vi "配置初始化.vi"(8 "error in (no error)":errorcluster) -> (0 "error out":errorcluster)   [LabVIEW 2016, in "斯坦道总氮.lvlib"]
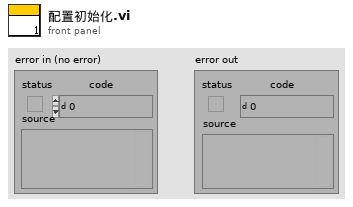
[diagram p1: front panel]
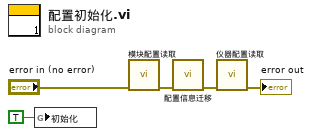
[diagram p0: block diagram]
diagram:
  n1 = global write "VAR总磷总氮全局变量.vi" "初始化"(TRUE ("内部初始化")) -> ()
  n2 = call "模块配置读取.vi"("error in (no error)"="error in (no error)") -> ("error out"=w4:errorcluster)  [unwired: 10 in]
  n3 = call "配置信息迁移.vi"("error in (no error)"=w4) -> ("error out"=w5:errorcluster)  [unwired: 10 in]
  n4 = call "仪器配置读取.vi"("error in (no error)"=w5) -> ("error out"=→"error out":errorcluster)  [unwired: 10 in]
